vi "Subpanel.vi"() -> ()   [LabVIEW 2013]
uses:
  GitHome/Tools/Laundry/Washer Soft Load Box/type defs/ERD_Always_Show.ctl
panel:
  out "data":T1
  in  "vi path":path=path "C:/GitHome/Tools/Laundry/Washer Soft Load Box/Laundry SLB Main.vi"
  in  "stop 2":bool
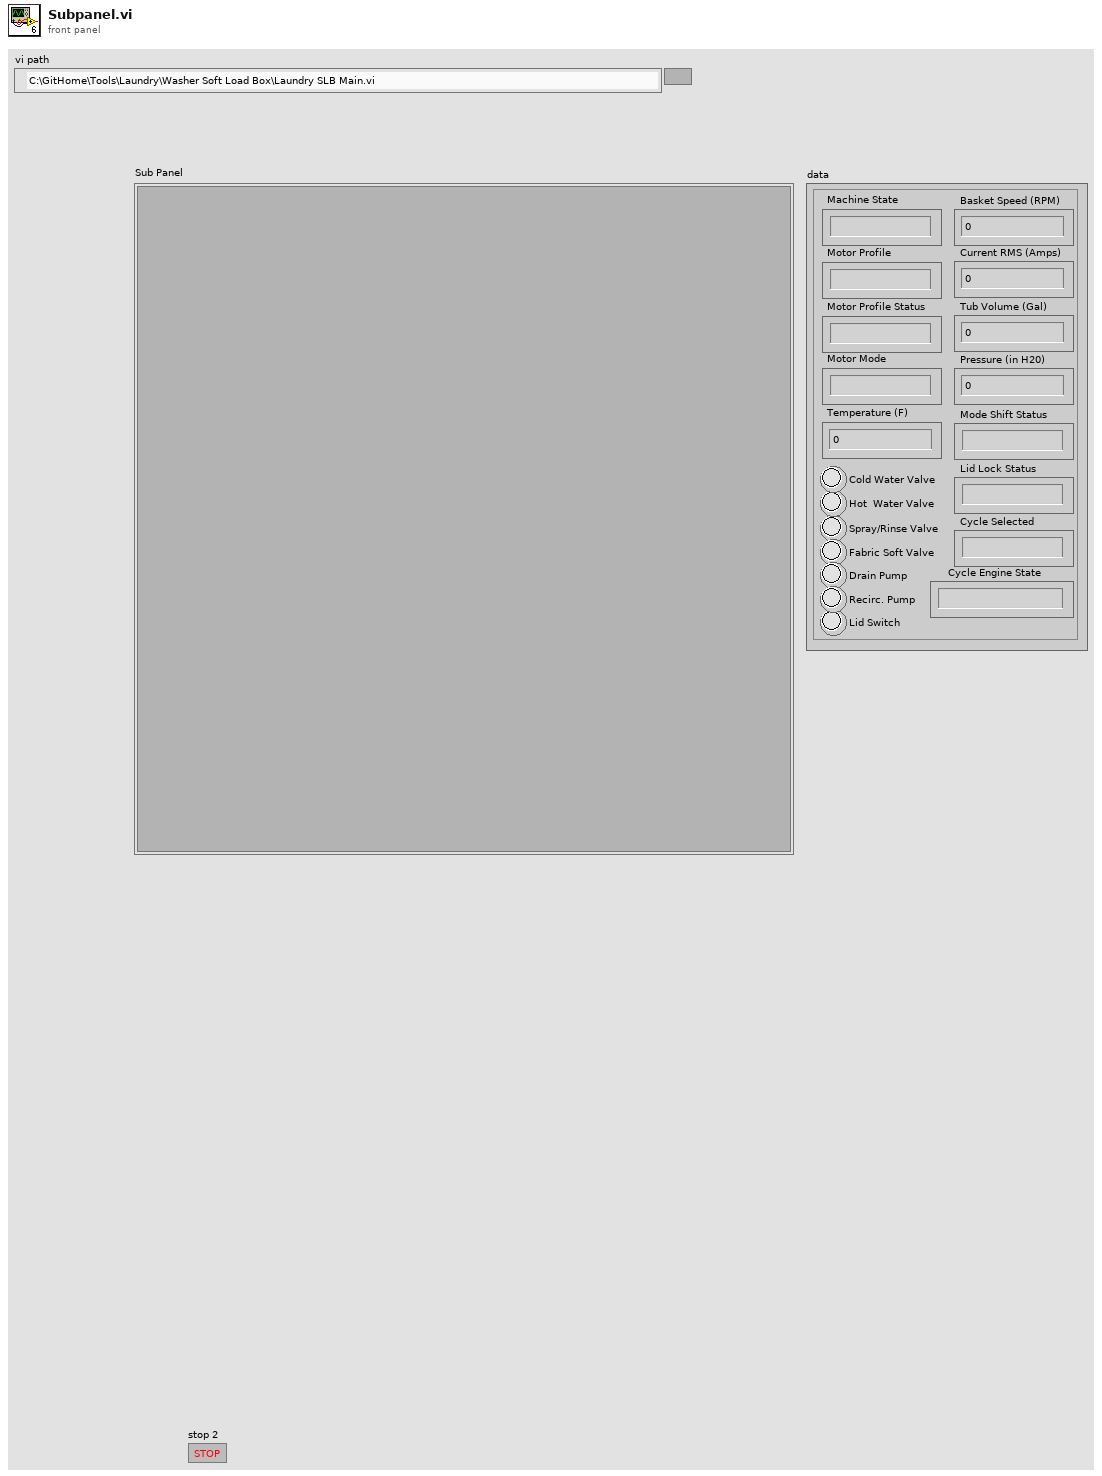
[diagram p1: front panel]
types:
  T1 = typedef "ERD_Always_Show.ctl" = cluster{"Basket Speed (RPM)":u16, "Machine State":string, "Tub Volume (Gal)":dbl, "Pressure (in H20)":dbl, "Motor Profile":string, "Motor Profile Status":string, "Temperature (F)":dbl, "Lid Switch ":bool, "Current RMS (Amps)":dbl, "Cycle Selected":string, "Lid Lock Status":string, "Mode Shift Status":string, "Spray/Rinse Valve":bool, "Fabric Soft Valve":bool, "Drain Pump":bool, "Recirc. Pump":bool, "Cycle Engine State":string, "Motor Mode":string, "Hot  Water Valve":bool, "Cold Water Valve":bool}
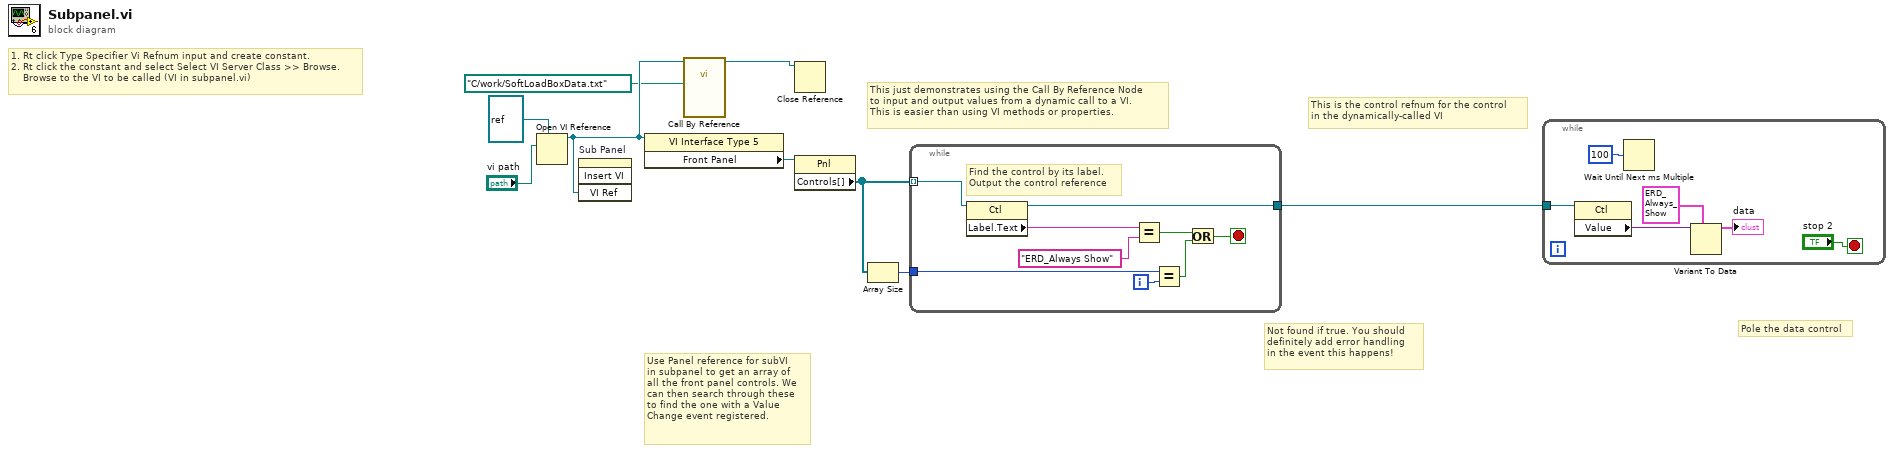
[diagram p0: block diagram]
diagram:
  # "Pole the data control"
  # "Use Panel reference for subVI\nin subpanel to get an array of\nall the front panel controls. We\ncan then search through these\nto find the one with a Value\nChange event registered."
  # "This is the control refnum for the control\nin the dynamically-called VI"
  # "This just demonstrates using the Call By Reference Node\nto input and output values from a dynamic call to a VI.\nThis is easier than using VI methods or properties."
  # "Not found if true. You should\ndefinitely add error handling\nin the event this happens!"
  # "1. Rt click Type Specifier Vi Refnum input and create constant.\n2. Rt click the constant and select Select VI Server Class >> Browse.\n    Browse to the VI to be called (VI in subpanel.vi)"
  n1 = Open VI Reference(type specifier VI Refnum (for type only)=refnum<vi> refnum, vi path="vi path") -> (vi reference=w3:refnum<vi>)  [unwired: 4 in, 1 out]
  n2 = invoke on="Sub Panel" class="SubPanel" method="Insert VI"("VI Ref"=w3) -> ()  [unwired: 3 in, 4 out]
  n3 = property class="VI Interface Type 5"(reference=w3) -> ("Front Panel"=w7:refnum<vi>)  [unwired: 1 in, 2 out]
  n4 = call-by-ref "?"(reference=w3, "File Path Control"=path "C:/work/SoftLoadBoxData.txt") -> (reference out=w8:refnum<vi>)  [unwired: 16 in, 1 out]
  n5 = Close Reference(reference=w8) -> ()  [unwired: 1 in, 1 out]
  n6 = property class="Pnl"(reference=w7) -> ("Controls[]"=w6:refnum<vi>[])  [unwired: 1 in, 2 out]
  n7 = Array Size(array=w6) -> (size(s)=w5:i32)
  n8 = while {
    tunnel: w6 -> [w18] mode=indexing
    tunnel: w5 -> [w17]
    tunnel: [w11] -> w4
    i -> [w16]
    stop <- w12 stop-if-true
    # "Find the control by its label.\nOutput the control reference"
    n9 = property class="Ctl"(reference=w18) -> (reference out=w11:refnum<vi>, "Label.Text"=w10:string)  [unwired: 1 in, 1 out]
    n10 = Equal?(x=w10, y="ERD_Always Show") -> (x = y?=w14:bool)
    n11 = Equal?(x=w17, y=w16) -> (x = y?=w13:bool)
    n12 = Or(x=w14, y=w13) -> (x .or. y?=w12:bool)
  }
  n13 = while {
    tunnel: w4 -> [w21]
    stop <- "stop 2" stop-if-true
    n14 = property class="Ctl"(reference=w21) -> ("Value"=w22:variant)  [unwired: 1 in, 2 out]
    n15 = Wait Until Next ms Multiple(millisecond multiple=u32 100) -> ()  [unwired: 1 out]
    n16 = Variant To Data(type=T1 {"Basket Speed (RPM)"=0, "Machine State"="", "Tub Volume (Gal)"=0.0, "Pressure (in H20)"=0.0, "Motor Profile"="", "Motor Profile Status"="", "Temperature (F)"=0.0, "Lid Switch "=FALSE, "Current RMS (Amps)"=0.0, "Cycle Selected"="", "Lid Lock Status"="", "Mode Shift Status"="", "Spray/Rinse Valve"=FALSE, "Fabric Soft Valve"=FALSE, "Drain Pump"=FALSE, "Recirc. Pump"=FALSE, "Cycle Engine State"="", "Motor Mode"="", "Hot  Water Valve"=FALSE, "Cold Water Valve"=FALSE} ("ERD_Always Show"), Variant=w22) -> (data=→"data":T1)  [unwired: 1 in, 1 out]
  }
